vi "Configure Channels.vi"(8 "error in":errorcluster, 11 "SDS1022 Base CFG in":refnum<class "SDS1022 Base CFG.lvclass">) -> (0 "error out":errorcluster, 3 "SDS1022 Base CFG out":refnum<class "SDS1022 Base CFG.lvclass">)   [LabVIEW 2023, in "OWON SDS1022.lvlib" / "SDS1022 Base CFG.lvclass"]
uses:
  SDS1022 Base CFG.lvclass
  HAL/Configuration Base/Configuration Base.lvclass/Configuration Base.ctl
  d33ed5e0-8481-4ea4-95cf-eb84cdcdc04c.vi
  aaa9d92d-73bc-46b3-bb81-b3bc91fdc2b4.vi
  <vilib>/JDP Science/JSONtext/Find Item.vi
  <vilib>/JDP Science/JSONtext/Next JSON Value.vi
  <vilib>/JDP Science/JSONtext/String Subset.vi
  <vilib>/JDP Science/JSONtext/Parsing/Advance past next JSON Value (inlined COPY).vi
  <vilib>/JDP Science/JSONtext/Parsing/Advance past whitespace.vi
  <vilib>/JDP Science/JSONtext/Parsing/Advance past String.vi
  <vilib>/JDP Science/JSONtext/Parsing/Advance past Number.vi
  <vilib>/JDP Science/JSONtext/Parsing/Advance past Line Ending.vi
  <vilib>/JDP Science/JSONtext/Parsing/Parse Full Path or Item Name.vi
  <vilib>/JDP Science/JSONtext/Parsing/Advance past Array.vi
  <vilib>/JDP Science/JSONtext/Parsing/Advance past Object.vi
  <vilib>/JDP Science/JSONtext/support/Error Cluster From Code.vi
  <vilib>/JDP Science/JSONtext/Offset/Find Item Locations by Path.vi
  <vilib>/JDP Science/JSONtext/JSON text to Variant.vi
  <vilib>/Utility/error.llb/Error Cluster From Error Code.vi
  <vilib>/JDP Science/JSONtext/LVClass Serializer/JSONtext LVClass Serializer.lvclass
  <vilib>/ErrorRing/Error Ring.xnode
  SDS1022 Base CFG.lvclass/SDS1022 Base CFG.ctl
  HAL/Configuration Base/Configuration Base.lvclass
  <instrlib>/OWON SDS1022/OWON SDS1022 Driver.lvlib
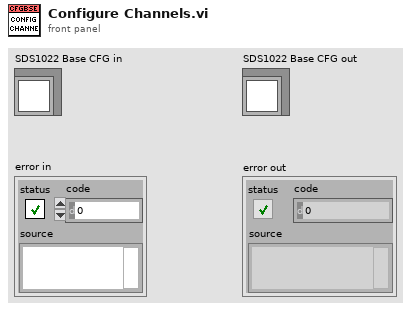
[diagram p1: front panel]
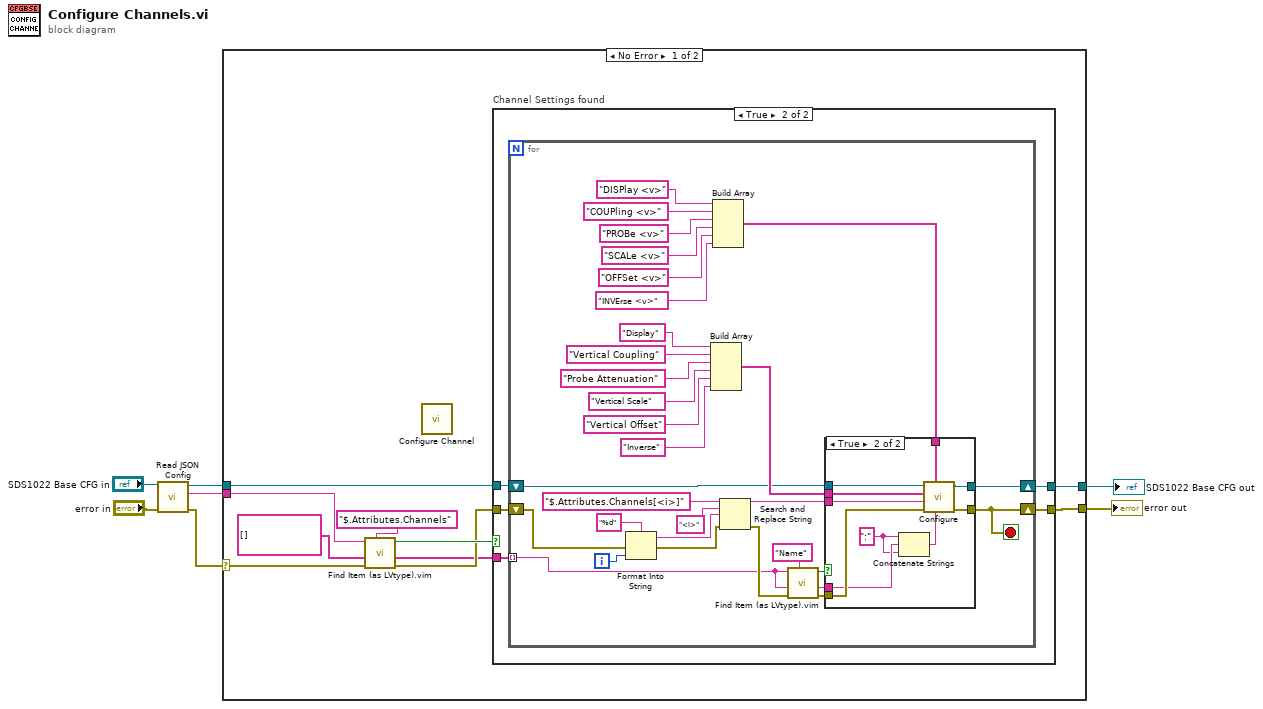
[diagram p0: block diagram]
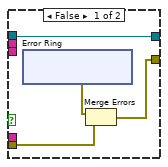
[diagram p3: hidden frame]
diagram:
  n1 = call "Read JSON Config.vi"("error in"="error in", "object in"="SDS1022 Base CFG in") -> ("error out"=w1:errorcluster, "<JSON>Config"=w5:string, "object out"=w4:refnum<class "SDS1022 Base CFG.lvclass">)  [unwired: 7 in]
  n2 = case shown="No Error" w1 {
    selector: w1 -> [w9 w76]
    tunnel: w5 -> [w16 _]
    tunnel: w4 -> [w12 w75]
    tunnel: [w11 w75] -> w3
    tunnel: [w10 w76] -> w2
    frame No Error {
      n3 = call "Find Item (as LVtype).vim"("$Path or Item Name"="$.Attributes.Channels", "error in (no error)"=w9, "Data Type and Default Value"=string[] [], "JSON"=w16) -> ("error out"=w14:errorcluster, "Data"=w13:string[], "Found"=w15:bool)  [unwired: 4 in, 1 out]
      n4 = call <instrlib>:"Configure Channel.vi"() -> ()  [unwired: 14 in, 2 out]
      n5 = case "Channel Settings found" shown="True" w15 {
        tunnel: w13 -> [_ w24]
        tunnel: w14 -> [w19 w23]
        tunnel: w12 -> [w18 w22]
        tunnel: [w19 w21] -> w10
        tunnel: [w18 w20] -> w11
        frame False {
        }
        frame True {
          n6 = for {
            tunnel: w24 -> [w25] mode=indexing
            shift-right: [w26] -> w21
            shift-left: w23 -> [w33]
            shift-right: [w40] -> w20
            shift-left: w22 -> [w48]
            i -> [w37]
            stop <- w26 stop-if-true
            n7 = Format Into String(format string="%d", error in=w33, w37) -> (resulting string=w34:string, error out=w32:errorcluster)  [unwired: 1 in]
            n8 = Build Array("Display" ("element"), "Vertical Coupling", "Probe Attenuation" ("element"), "Vertical Scale" ("element"), "Vertical Offset", "Inverse") -> (w49:string[])
            n9 = Build Array("DISPlay <v>" ("element"), "COUPling <v>", "PROBe <v>", "SCALe <v>", "OFFSet <v>", "INVErse <v>") -> (w41:string[])
            n10 = Search and Replace String(input string="$.Attributes.Channels[<i>]" ("$Path or Item Name"), search string="<i>", replace string=w34, error in=w32) -> (result string=w38:string, error out=w30:errorcluster)  [unwired: 4 in, 2 out]
            n11 = call "Find Item (as LVtype).vim"("$Path or Item Name"="Name", "error in (no error)"=w30, "Data Type and Default Value"=w25, "JSON"=w25) -> ("error out"=w29:errorcluster, "Data"=w28:string, "Found"=w27:bool)  [unwired: 4 in, 1 out]
            n12 = case shown="True" w27 {
              tunnel: w49 -> [_ w74]
              tunnel: w48 -> [w56 w73]
              tunnel: w41 -> [_ w72]
              tunnel: [w57 w71] -> w26
              tunnel: [w56 w70] -> w40
              tunnel: w38 -> [_ w69]
              tunnel: w29 -> [w59 w68]
              tunnel: w28 -> [_ w67]
              frame False {
                n13 = xnode "Error Ring"() -> ("error out"=w58:errorcluster)
                n14 = Merge Errors(w58, w59) -> (w57:errorcluster)
              }
              frame True {
                w65 = ":" ("string")
                n15 = Concatenate Strings(w65, w67, w65) -> (w66:string)
                n16 = call "Configure.vi"("CMD Prefix"=w66, "CMDs"=w72, "error in"=w68, "JSON Settings Path"=w69, "JSON Keys"=w74, "object in"=w73) -> ("error out"=w71:errorcluster, "object out"=w70:refnum<class "SDS1022 Base CFG.lvclass">)  [unwired: 4 in]
              }
            }
          }
        }
      }
    }
    frame Error {
    }
  }
  "SDS1022 Base CFG out" <- w3
  "error out" <- w2
